vi "PlayerInfoBroadcaster.vi"(0 "PlayerInfoMap":T1(c390)) -> ()   [LabVIEW 2025]
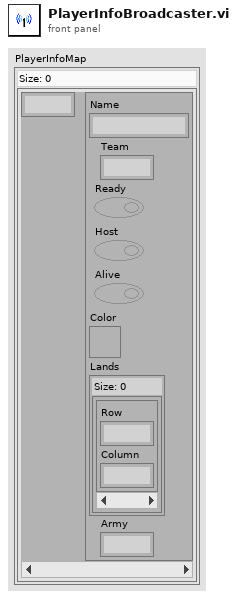
[diagram p1: front panel]
types:
  T1 = map{u32, cluster{"Name":string, "Team":u8, "Ready":bool, "Host":bool, "Alive":bool, "Color":u32, "Lands":set{cluster{"Row":u32, "Column":u32}}, "Army":u32}}
  T2 = cluster{"ID":u32, "Name":string, "Team":u8, "Ready":bool, "Host":bool, "Alive":bool, "Color":u32, "Lands":set{cluster{"Row":u32, "Column":u32}}, "Army":u32}[]
  T3 = cluster{"ID":u32, "Name":string, "Team":u8, "Ready":bool, "Host":bool, "Alive":bool, "Color":u32, "Lands":set{cluster{"Row":u32, "Column":u32}}, "Army":u32}
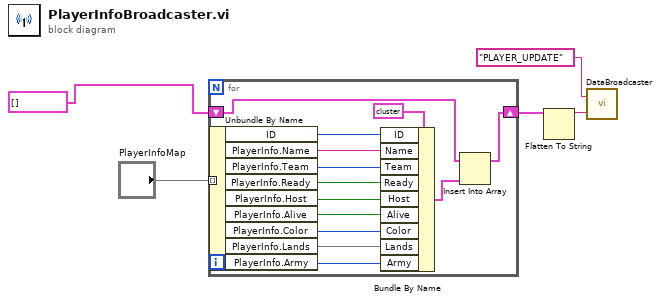
[diagram p0: block diagram]
diagram:
  n1 = for {
    tunnel: "PlayerInfoMap" -> [w17] mode=indexing
    shift-right: [w19] -> w5
    shift-left: T2 [] ("PlayerInfoArray") -> [w18]
    n2 = Unbundle By Name(w17) -> ("ID"=w15:u32, "PlayerInfo.Name"=w14:string, "PlayerInfo.Team"=w13:u8, "PlayerInfo.Ready"=w12:bool, "PlayerInfo.Host"=w11:bool, "PlayerInfo.Alive"=w10:bool, "PlayerInfo.Color"=w9:u32, "PlayerInfo.Lands"=w8:set{cluster{"Row":u32, "Column":u32}}, "PlayerInfo.Army"=w7:u32)
    n3 = Bundle By Name(cluster=T3 {"ID"=0, "Name"="", "Team"=0, "Ready"=FALSE, "Host"=FALSE, "Alive"=FALSE, "Color"=0, "Lands"={}, "Army"=0} ("PlayerInfo"), "ID"=w15, "Name"=w14, "Team"=w13, "Ready"=w12, "Host"=w11, "Alive"=w10, "Color"=w9, "Lands"=w8, "Army"=w7) -> (w6:T3)
    n4 = Insert Into Array(array=w18, new element=w6) -> (w19:T2)  [unwired: 1 in]
  }
  n5 = Flatten To String(anything=w5) -> (data string=w4:string)  [unwired: 3 in, 2 out]
  n6 = call "DataBroadcaster.vi"("Data"=w4, "Action"="PLAYER_UPDATE") -> ()
